vi "elvisv1_2.vi"(0 "Device Name":tag="Dev1", 1 "Amplitude":dbl, 2 "DC Offset":dbl, 3 "Frequency":dbl, 4 "Waveform Type":enum16{"Sine", "Triangular", "Square"}(ring), 5 "Sample Rate (Hz)":dbl=100000.0 caption="Sample rate (S/s)" min=0.0 step=1000000.0 format="%#_4p", 6 "Record Length":i32=2000 caption="Record length" min=5 max=75000000 step=1 format="%#.9p", 7 "Acquire":u16(ring)=10178 items=["N Samples"=10178, "Continuously"=10123], 8 "ChA_Source":u16(ring) caption="Source" items=["CH0", "CH1", "CH2", "CH3"], 9 "ChB_Source":u16(ring) caption="Source" items=["CH4", "CH5", "CH6", "CH7"], 10 "ChA Coupling":u16(ring) caption="Coupling" items=["DC", "AC"], 11 "ChB_ Coupling":u16(ring) caption="Coupling" items=["DC", "AC"], 12 "ChA Range":dbl caption="Range", 13 "ChB Range":dbl caption="Range", 14 "ChA Offset":dbl caption="Offset", 15 "ChB Offset":dbl caption="Offset", 16 "Trigger Source":u16(ring) caption="Source" items=["Immediate", "TRIGGER", "SYNC_OUT", "CH A", "CH B"], 17 "Trigger Type":u16(ring) caption="Type" items=["Digital", "Analog"], 18 "Slope":i32(ring) items=["Positive", "Negative"], 19 "setupID":i32, 27 "input_FG_Connection":u8) -> (22 "interleaved array":dbl[](array[numeric]))   [LabVIEW 2010]
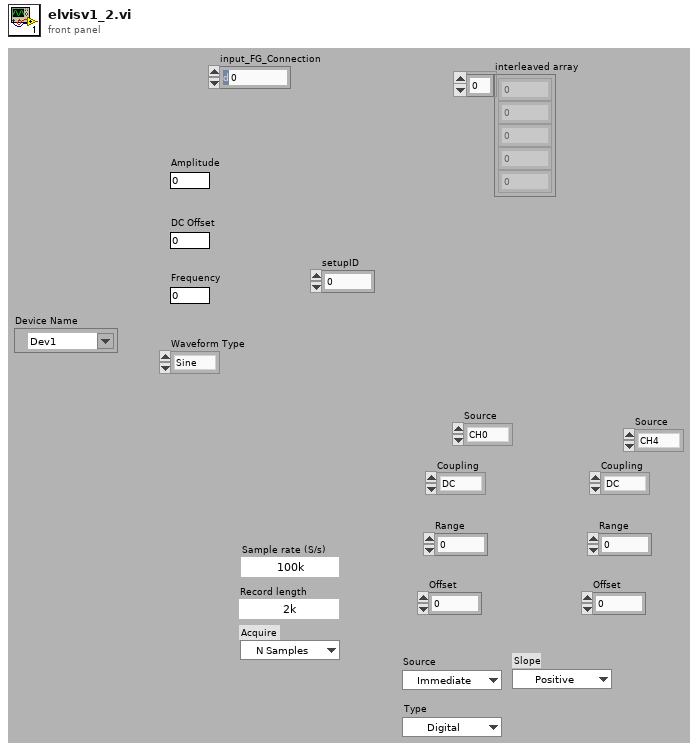
[diagram p1: front panel]
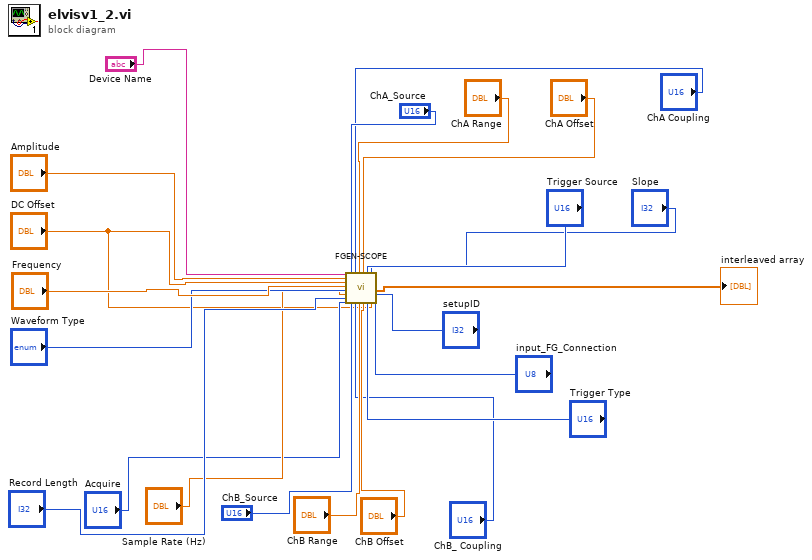
[diagram p0: block diagram]
diagram:
  n1 = call "FGEN-SCOPE.vi"("Device Name"="Device Name", "Amplitude"="Amplitude", "DC Offset"="DC Offset", "Frequency"="Frequency", "Waveform Type"="Waveform Type", "Sample Rate (Hz)"="Sample Rate (Hz)", "Record Length"="Record Length", "Acquire"="Acquire", "ChA_Source"="ChA_Source", "ChB_Source"="ChB_Source", "ChA Coupling"="ChA Coupling", "ChB_ Coupling"="ChB_ Coupling", "ChA Range"="ChA Range", "ChB Range"="ChB Range", "ChA Offset"="ChA Offset", "ChB Offset"="ChB Offset", "Trigger Source"="Trigger Source", "Trigger Type"="Trigger Type", "Slope"="Slope", "Level"="DC Offset", "SetupID"="setupID", "input_FG_Connection"="input_FG_Connection") -> ("interleaved array"=→"interleaved array":dbl[])  [unwired: 4 in, 1 out]
